vi "Actor Core.vi"(8 "error in":errorcluster, 11 "Main ViewManager In":refnum<class "Navigation ViewManager.lvclass">) -> (0 "error out":errorcluster, 3 "Actor out":refnum<class "Actor.lvclass">)   [LabVIEW 2019, in "Navigation ViewManager.lvclass"]
doc: "(<B>Filename</B>: Actor Framework.lvlib:Actor.lvclass:Actor Core.vi)\n\nReceives messages to the actor, reacts to them, and initiates any error handling that may shut the actor down.\n\nDescendant classes may override this VI to append parallel tasks for the actor to complete while it handles messages. Overrides use the Call Parent Method node.\n\n<License>\nCopyright © 2017 Composed Systems, LLC | All rights reserved\nwww.composed.io\n\nAuthor: Ethan Stern <ethan.stern@composed.io>\n\nThis software is provided \"AS IS\" WITHOUT WARRANTIES, either express or implied, AND IS FOR EDUCATIONAL PURPOSES ONLY.\n</License>"
uses:
  <vilib>/gpm_packages/@cs/Car-wash/Source/Process Builder ViewManager/Navigation ViewManager.lvclass
  <vilib>/ActorFramework/Actor/Actor.lvclass
  <vilib>/gpm_packages/@cs/Car-wash/Source/Process Builder ViewManager/Navigation ViewManager.lvclass/Navigation ViewManager.ctl
  <vilib>/gpm_packages/@cs/mva-viewable/Source/IViewManager/IViewManager/IViewManager.lvclass
  <vilib>/gpm_packages/@cs/mva-viewable/Source/IViewable/ProtectedSubpanel/ProtectedSubpanel.lvclass
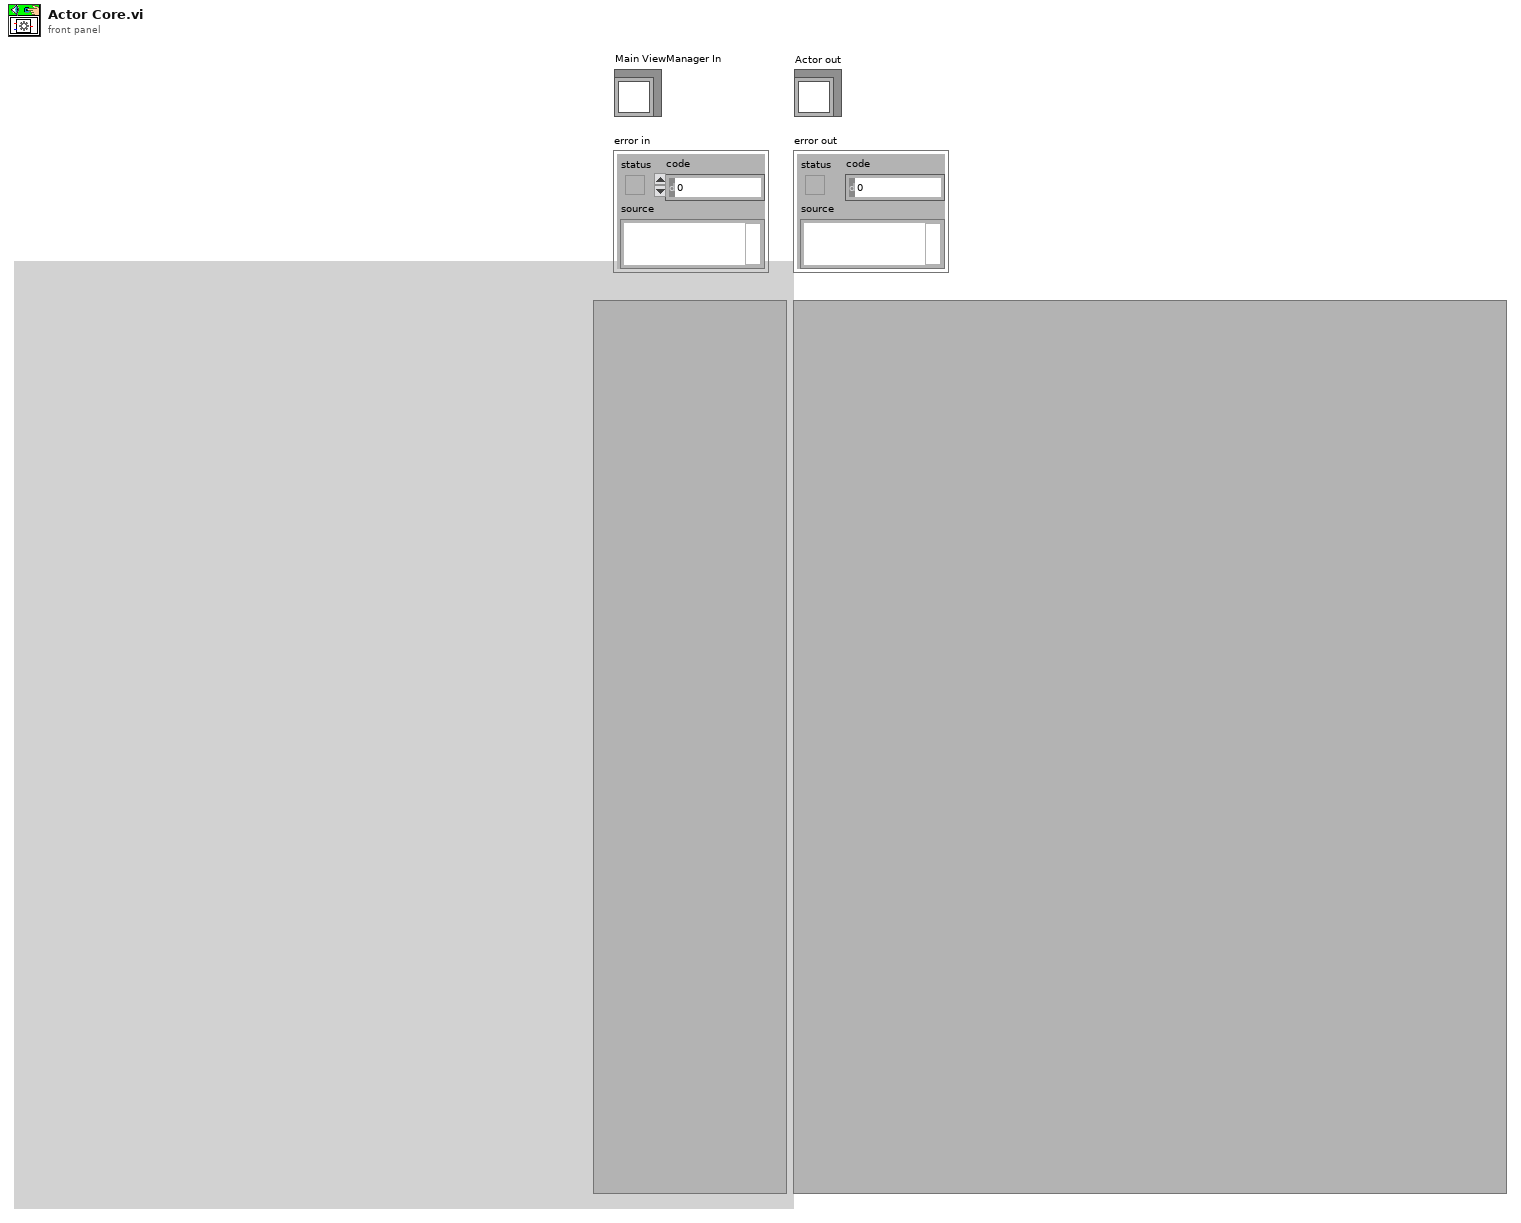
[diagram p1: front panel]
types:
  T1 = typedef "IViewable.lvlib/ProtectedSubpanel.lvclass/Protected Subpanel Reference.ctl" = refnum<data-value>
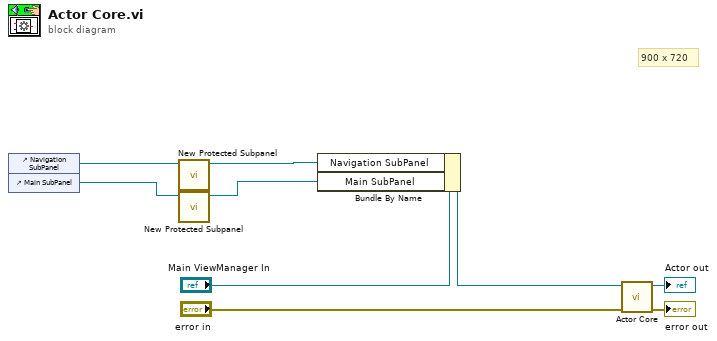
[diagram p0: block diagram]
diagram:
  # "900 x 720"
  n1 = control-ref of="Navigation SubPanel"() -> (w6:refnum<vi>)
  n2 = control-ref of="Main SubPanel"() -> (w7:refnum<vi>)
  n3 = call <vilib>:"New Protected Subpanel.vi"("SubPnl Refnum"=w6) -> ("Protected Subpanel"=w5:T1)  [unwired: 9 in, 1 out]
  n4 = call <vilib>:"New Protected Subpanel.vi"("SubPnl Refnum"=w7) -> ("Protected Subpanel"=w4:T1)  [unwired: 9 in, 1 out]
  n5 = Bundle By Name(cluster="Main ViewManager In", "Navigation SubPanel"=w5, "Main SubPanel"=w4) -> (w2:refnum<class "Navigation ViewManager.lvclass">)
  n6 = call-parent "Actor Core.vi"("error in"="error in", "IViewable In"=w2) -> ("error out"=→"error out":errorcluster, "Actor out"=→"Actor out":refnum<class "Actor.lvclass">)  [unwired: 8 in]
